vi "Get Departments.vi"(8 "error in (no error)":errorcluster, 11 "CalAttendance in":refnum<class "CalAttendance.lvclass">) -> (0 "error out":errorcluster, 2 "Departments(\"\")":string[](array[string]), 3 "CalAttendance out":refnum<class "CalAttendance.lvclass">)   [LabVIEW 2015, in "Admin_Actor.lvlib" / "CalAttendance.lvclass"]
uses:
  CalAttendance.lvclass
  CalAttendance.lvclass/CalAttendance.ctl
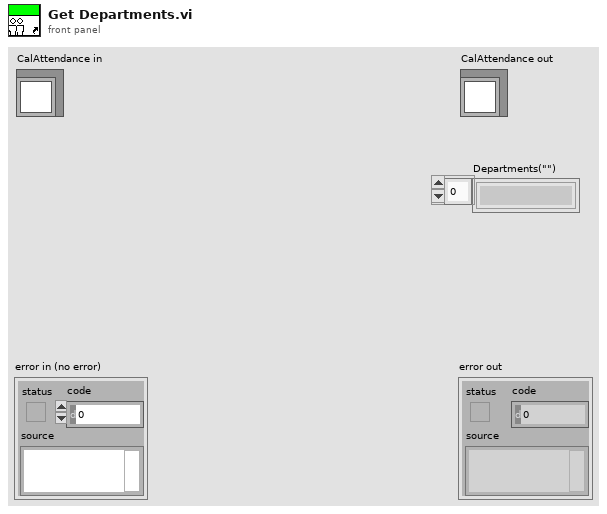
[diagram p1: front panel]
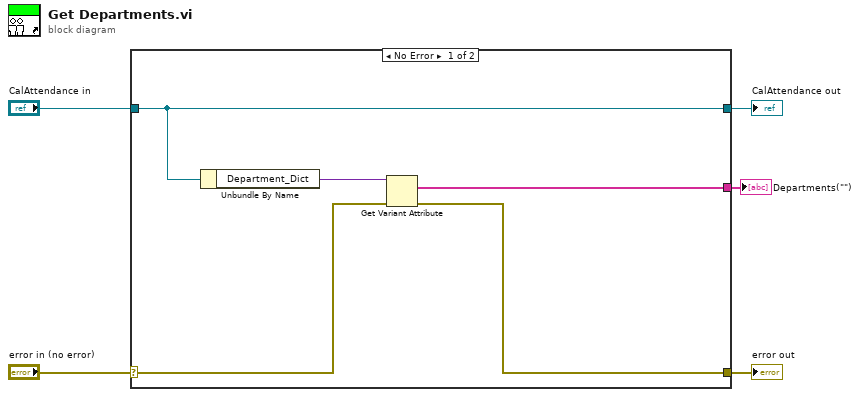
[diagram p0: block diagram]
diagram:
  n1 = case shown="No Error" "error in (no error)" {
    selector: "error in (no error)" -> [w7 w12]
    tunnel: [w6 w12] -> w4
    tunnel: [w10 w11] -> w2
    tunnel: "CalAttendance in" -> [w10 w11]
    tunnel: [w8 _] -> w1
    frame No Error {
      n2 = Unbundle By Name(w10) -> ("Department_Dict"=w9:variant)
      n3 = Get Variant Attribute(Variant=w9, error in=w7) -> (names=w8:string[], error out=w6:errorcluster)  [unwired: 2 in, 2 out]
    }
    frame Error {
    }
  }
  "error out" <- w4
  "CalAttendance out" <- w2
  "Departments(\"\")" <- w1
